vi "Close.vi"(8 "error in (no error)":errorcluster, 11 "Stand in":refnum<class "Stand.lvclass">) -> (0 "error out":errorcluster)   [LabVIEW 2019, in "Stand.lvclass"]
uses:
  Stand.lvclass
  C:/Users/ANENKOV_V1/Desktop/src/Proccess_class/Proccess.lvclass
  C:/Users/ANENKOV_V1/Desktop/src/Device_class/Device.lvclass
  MessageAMC_class/MessageAMC.lvclass
  Device_class/Device.lvclass/Device.ctl
  Proccess_class/Proccess.lvclass/Proccess.ctl
  Stand.lvclass/Stand.ctl
  NeedleValve_class/NeedleValve.lvclass
  FPGA_API_class/FPGA API.lvclass
  Proccess_class/Proccess.lvclass
  Logger_class/Logger.lvclass
  Device_class/Device.lvclass
  Modbus_class/ModbusSp.lvclass
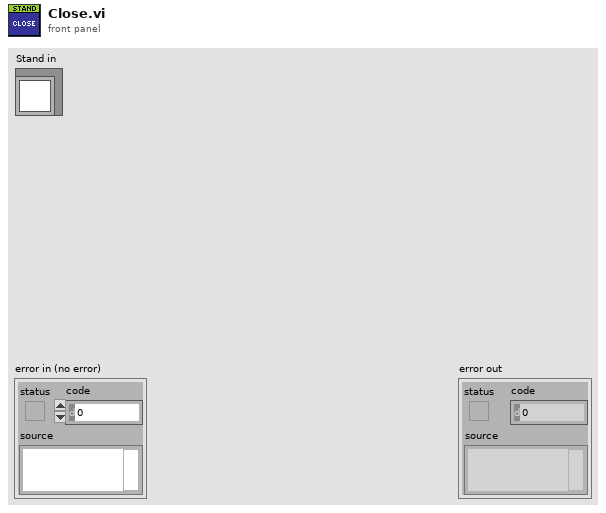
[diagram p1: front panel]
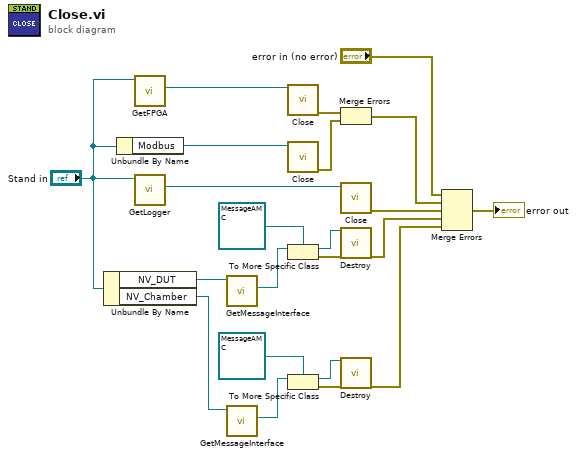
[diagram p0: block diagram]
diagram:
  n1 = Unbundle By Name("Stand in") -> ("NV_DUT"=w4:refnum<class "NeedleValve.lvclass">, "NV_Chamber"=w3:refnum<class "NeedleValve.lvclass">)
  n2 = Unbundle By Name("Stand in") -> ("Modbus"=w2:refnum<class "ModbusSp.lvclass">)
  n3 = call "GetFPGA.vi"("Device in"="Stand in") -> ("FPGA API.lvclass"=w6:refnum<class "FPGA API.lvclass">)  [unwired: 10 in]
  n4 = call "GetLogger.vi"("Proccess in"="Stand in") -> ("Logger"=w20:refnum<class "Logger.lvclass">)  [unwired: 10 in]
  n5 = call "GetMessageInterface.vi"("Device in"=w4) -> ("MessageInterface"=w16:refnum<class "MessageInterface.lvclass">)  [unwired: 10 in]
  n6 = call "GetMessageInterface.vi"("Device in"=w3) -> ("MessageInterface"=w8:refnum<class "MessageInterface.lvclass">)  [unwired: 10 in]
  n7 = call-dynamic "Close.vi"("FPGA API in"=w6) -> ("error out"=w17:errorcluster)  [unwired: 13 in, 1 out]
  n8 = call "Close.vi"("ModbusSp in"=w2) -> ("error out"=w1:errorcluster)  [unwired: 9 in, 1 out]
  n9 = To More Specific Class(target class=refnum<class "MessageAMC.lvclass"> refnum ("reference in"), reference=w16) -> (specific class reference=w14:refnum<class "MessageAMC.lvclass">, error out=w13:errorcluster)  [unwired: 1 in]
  n10 = To More Specific Class(target class=refnum<class "MessageAMC.lvclass"> refnum ("reference in"), reference=w8) -> (specific class reference=w10:refnum<class "MessageAMC.lvclass">, error out=w11:errorcluster)  [unwired: 1 in]
  n11 = Merge Errors(w17, w1) -> (w18:errorcluster)
  n12 = call "Close.vi"("Logger in"=w20) -> ("error out"=w19:errorcluster)  [unwired: 9 in, 1 out]
  n13 = call-dynamic "Destroy.vi"("reference in"=w14, "error in (no error)"=w13) -> ("error out"=w12:errorcluster)  [unwired: 16 in, 1 out]
  n14 = call-dynamic "Destroy.vi"("reference in"=w10, "error in (no error)"=w11) -> ("error out"=w7:errorcluster)  [unwired: 16 in, 1 out]
  n15 = Merge Errors("error in (no error)", w18, w19, w12, w7) -> (→"error out":errorcluster)
